vi "addBooleanElement.vi"(7 "Name":string, 8 "error in (no error)":errorcluster, 9 "Value":bool, 10 "Replace? (false)":bool, 11 "tBSONDocument in":refnum<class "tBSONDocument.lvclass">) -> (0 "error out":errorcluster, 3 "tBSONDocument out":refnum<class "tBSONDocument.lvclass">)   [LabVIEW 2013, in "BSON.lvlib" / "tBSONDocument.lvclass"]
doc: "Adds a boolean to a BSON document."
uses:
  tBSONDocument.lvclass
  BSONElements/tBSONBoolean/tBSONBoolean.lvclass
  tBSONElement/tBSONElement.lvclass
  tBSONElement/setName.vi
  BSONElements/tBSONBoolean/setValue.vi
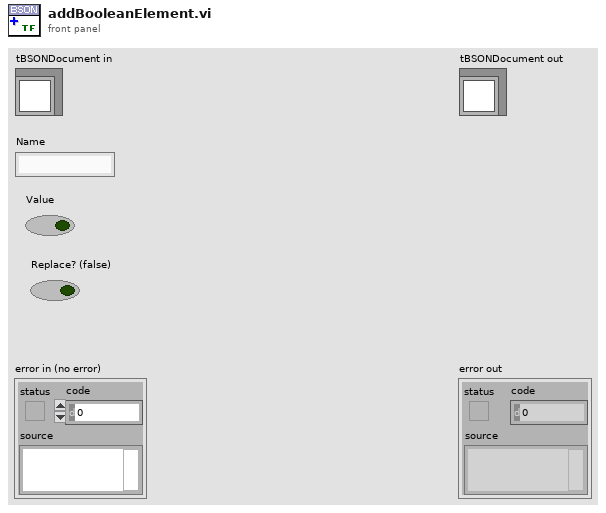
[diagram p1: front panel]
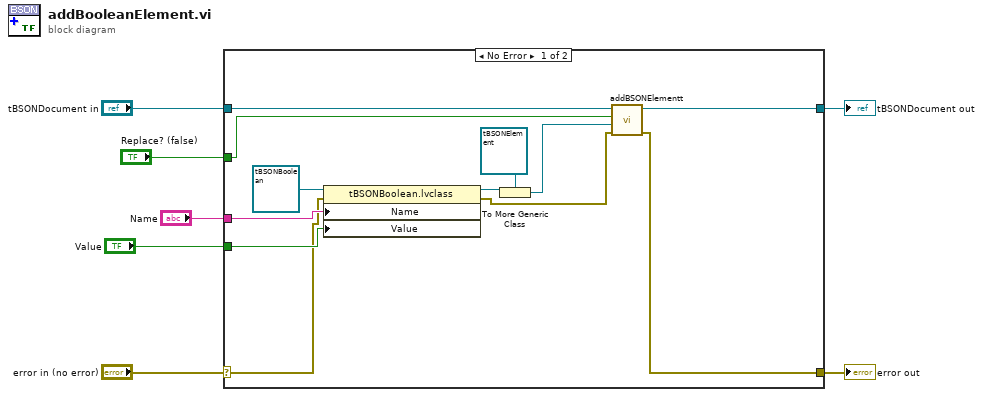
[diagram p0: block diagram]
diagram:
  n1 = case shown="No Error" "error in (no error)" {
    selector: "error in (no error)" -> [w13 w21]
    tunnel: [w10 w21] -> w6
    tunnel: [w9 w20] -> w4
    tunnel: "tBSONDocument in" -> [w14 w20]
    tunnel: "Name" -> [w18 _]
    tunnel: "Value" -> [w17 _]
    tunnel: "Replace? (false)" -> [w8 _]
    frame No Error {
      n2 = property class="tBSONBoolean.lvclass"(reference=refnum<class "tBSONBoolean.lvclass"> refnum ("BSON.lvlib:tBSONBoolean.lvclass"), error in=w13, "Name"=w18, "Value"=w17) -> (reference out=w16:refnum<class "tBSONBoolean.lvclass">, error out=w12:errorcluster)
      n3 = To More Generic Class(target class=refnum<class "tBSONElement.lvclass"> refnum ("BSON.lvlib:tBSONElement.lvclass"), reference=w16) -> (generic class reference=w11:refnum<class "tBSONElement.lvclass">)
      n4 = call "addBSONElementt.vi"("error in (no error)"=w12, "Element"=w11, "Replace? (false)"=w8, "tBSONDocument in"=w14) -> ("error out"=w10:errorcluster, "tBSONDocument out"=w9:refnum<class "tBSONDocument.lvclass">)  [unwired: 6 in]
    }
    frame Error {
    }
  }
  "error out" <- w6
  "tBSONDocument out" <- w4
